vi "test realtime main.vi"() -> ()   [LabVIEW 2012]
uses:
  GlobalVars.vi
panel:
  in  "Average N Reference Frames":dbl=1.0 min=1.0
  in  "Position Shift Limit (Microns)":dbl=3.0 min=0.0
  out "Out of Limits":bool
  in  "output cluster":T1
  out "Z":waveform(dbl)(graph)
  out "Y":waveform(dbl)(graph)
  out "X":waveform(dbl)(graph)
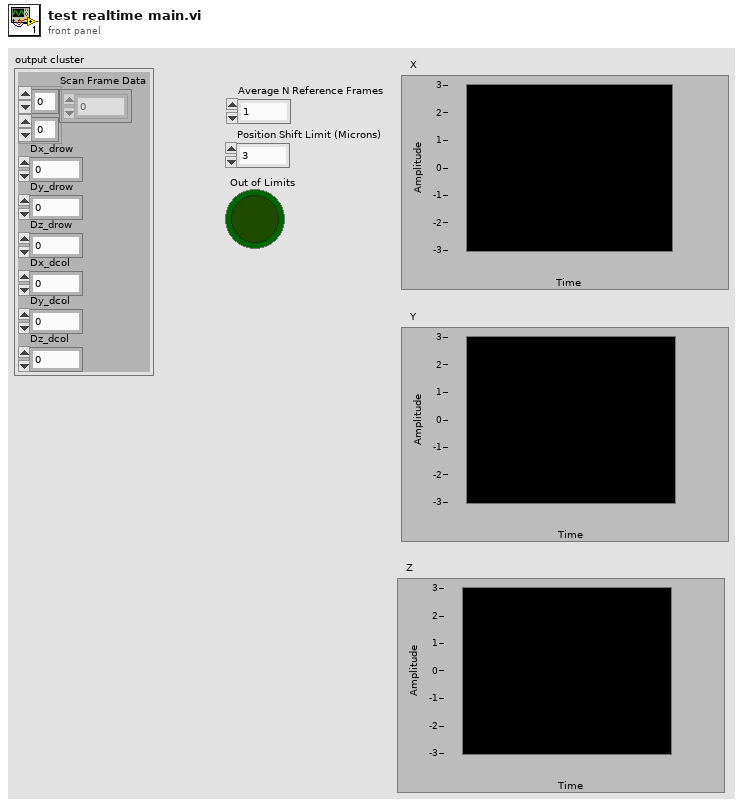
[diagram p1: front panel]
types:
  T1 = cluster{"Scan Frame Data":dbl[][], "Dx_drow":dbl, "Dy_drow":dbl, "Dz_drow":dbl, "Dx_dcol":dbl, "Dy_dcol":dbl, "Dz_dcol":dbl}
  T2 = cluster{"PMTChans":i32, "NumScanPlanes":i32, "ScanRows":i32, "ScanCols":i32, "NumSamples":i32}
  T3 = cluster{"Scan Frame Data":dbl[][], "Dx_drow":dbl, "Dy_drow":dbl, "Dz_drow":dbl, "Dx_dcol":dbl, "Dy_dcol":dbl, "Dz_dcol":dbl}[]
  T4 = cluster{"Scan Frame Data":dbl[][], dbl, dbl, dbl, dbl, dbl, dbl}
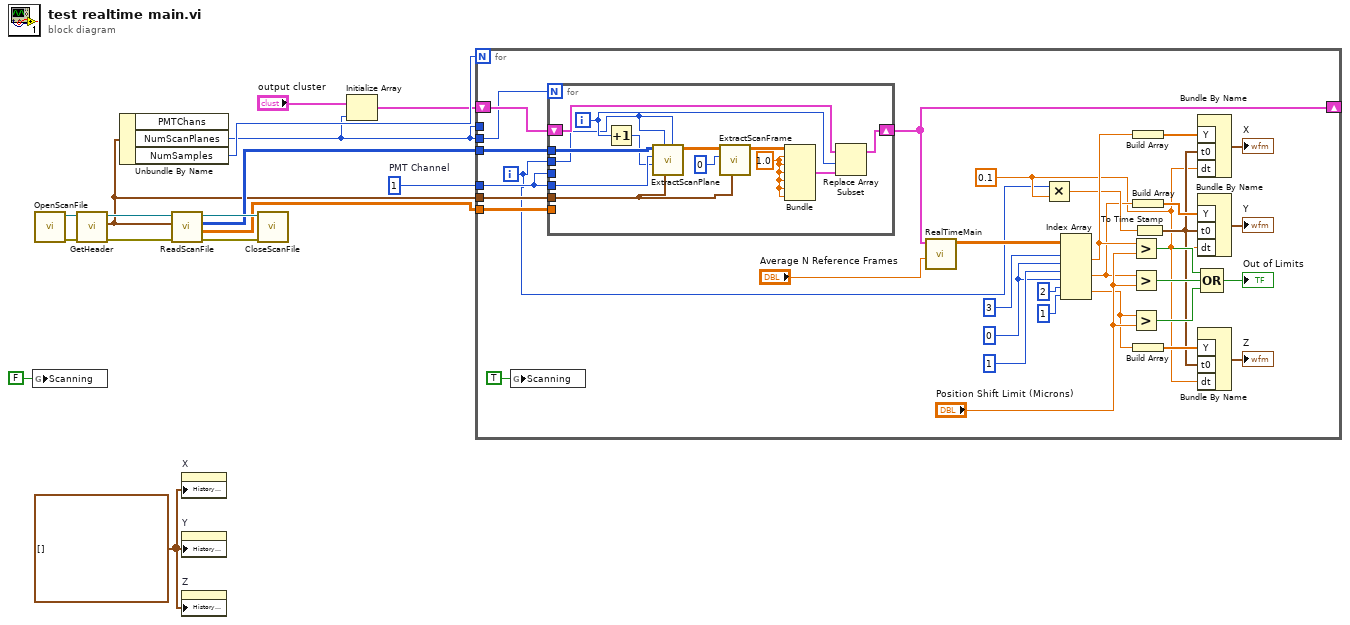
[diagram p0: block diagram]
diagram:
  w2 = waveform(dbl)[] [] ("History Data")
  w7 = 1  # PMT Channel
  n1 = global write "GlobalVars.vi" "Scanning"(FALSE ("Scanning")) -> ()
  n2 = call "OpenScanFile.vi"() -> ("error out"=w15:errorcluster, "refnum out"=w16:refnum<file>)  [unwired: 10 in]
  n3 = call "GetHeader.vi"("error in"=w15, "refnum in"=w16) -> ("error out"=w11:errorcluster, "Header"=w8:T2, "refnum out"=w14:refnum<file>)  [unwired: 6 in]
  n4 = Unbundle By Name(w8) -> ("NumScanPlanes"=w3:i32, "NumSamples"=w6:i32)  [unwired: 1 out]
  n5 = call "ReadScanFile.vi"("error in"=w11, "Header"=w8, "refnum in"=w14) -> ("error out"=w12:errorcluster, "Coordinate Data"=w9:dbl[][][][], "Scan Data"=w10:i32[][][][], "refnum out"=w13:refnum<file>)  [unwired: 5 in]
  n6 = property on="X" class="WFChart (strict)"("History Data"=w2) -> ()  [unwired: 2 in, 2 out]
  n7 = property on="Y" class="WFChart (strict)"("History Data"=w2) -> ()  [unwired: 2 in, 2 out]
  n8 = property on="Z" class="WFChart (strict)"("History Data"=w2) -> ()  [unwired: 2 in, 2 out]
  n9 = call "CloseScanFile.vi"("error in"=w12, "refnum"=w13) -> ()  [unwired: 9 in, 1 out]
  n10 = Initialize Array("output cluster", w3) -> (w4:T3)
  n11 = for {
    N: w6 -> [_]
    tunnel: w10 -> [w49]
    tunnel: w9 -> [w48]
    tunnel: w8 -> [w31]
    tunnel: w3 -> [w45]
    tunnel: w7 -> [w47]
    shift-right: [w44] -> _
    shift-left: w4 -> [w46]
    tunnel: w3 -> [_]
    i -> [w17]
    w19 = 0.1 ("dt")
    w39 = 0 ("disabled index (col)")
    n12 = global write "GlobalVars.vi" "Scanning"(TRUE ("Scanning")) -> ()
    n13 = for {
      N: w45 -> [_]
      tunnel: w49 -> [w62]
      tunnel: w47 -> [w61]
      tunnel: w48 -> [_]
      tunnel: w31 -> [w58]
      tunnel: w47 -> [_]
      tunnel: w17 -> [w52]
      shift-right: [w53] -> w44
      shift-left: w46 -> [w56]
      i -> [w54]
      w50 = 1.0
      n14 = Increment(x=w54) -> (x+1=w59:i32)
      n15 = call "ExtractScanPlane.vi"("End Frame"=w52, "Header"=w58, "Start Frame"=w52, "Scan Plane"=w59, "PMT Channel"=w61, "All Scan Data"=w62) -> ("Scan Plane Data"=w60:dbl[][][])  [unwired: 5 in]
      n16 = call "ExtractScanFrame.vi"("Header"=w58, "Scan Frame"=0, "Scan Plane Data"=w60) -> ("Scan Frame Data"=w57:dbl[][])  [unwired: 8 in]
      n17 = Bundle("Scan Frame Data"=w57, w50, w50, w50, w50, w50, w50) -> (w55:T4)  [unwired: 1 in]
      n18 = Replace Array Subset(array=w56, new element=w55, index=w54) -> (w53:T3)
    }
    n19 = call "RealTimeMain.vi"("For Reference (frames)"="Average N Reference Frames", "Motion Data"=w44) -> ("Array"=w34:dbl[][])  [unwired: 9 in]
    n20 = Multiply(x=w17, y=w19) -> (x*y=w24:dbl)
    n21 = Index Array(array=w34, index (row) #1=3 ("index (row)"), index (col) #1=w39, index (row) #2=1 ("index (row)"), index (col) #2=w39, index (row) #3=2 ("index (row)"), index (col) #3=1 ("disabled index (col)")) -> (element #1=w25:dbl, element #2=w21:dbl, element #3=w28:dbl)
    n22 = Greater?(x=w25, y="Position Shift Limit (Microns)") -> (0:w37:bool)
    n23 = Greater?(x=w21, y="Position Shift Limit (Microns)") -> (0:w36:bool)
    n24 = Greater?(x=w28, y="Position Shift Limit (Microns)") -> (0:w35:bool)
    n25 = Build Array(w25) -> (w26:dbl[])
    n26 = Build Array(w21) -> (w22:dbl[])
    n27 = Build Array(w28) -> (w29:dbl[])
    n28 = To Time Stamp(1:w24) -> (0:w20:timestamp)
    n29 = Bundle By Name("Y"=w26, "t0"=w20, "dt"=w19) -> (→"X":waveform(dbl))  [unwired: 1 in]
    n30 = Bundle By Name("Y"=w22, "t0"=w20, "dt"=w19) -> (→"Y":waveform(dbl))  [unwired: 1 in]
    n31 = Bundle By Name("Y"=w29, "t0"=w20, "dt"=w19) -> (→"Z":waveform(dbl))  [unwired: 1 in]
    n32 = Compound Arithmetic op=OR(w37, w36, w35) -> (→"Out of Limits":bool)
  }
